vi "___rate scan pruebas.vi"(6 "T Ventana":u32 format="%x", 7 "Espera acceso USB":u32, 8 "error in 2":errorcluster, 9 "Valor buscado scalers (5000)":u16, 10 "Sumador":u8, 11 "ftHandle_in 2":u32) -> (0 "error out 2":errorcluster, 1 "Scaler 3\nTH3,TH4,TH5":u16, 2 "Scaler 2\nTH0,TH1,TH2":u16, 3 "ftHandle_out 2":u32)   [LabVIEW 2009]
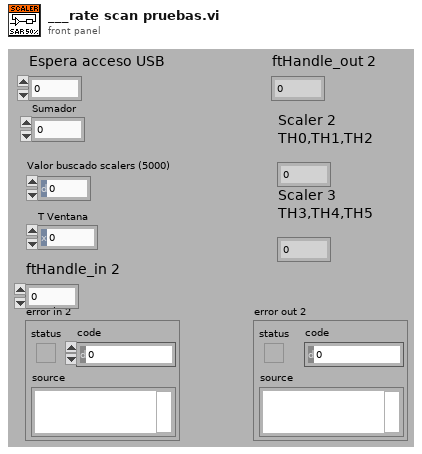
[diagram p1: front panel]
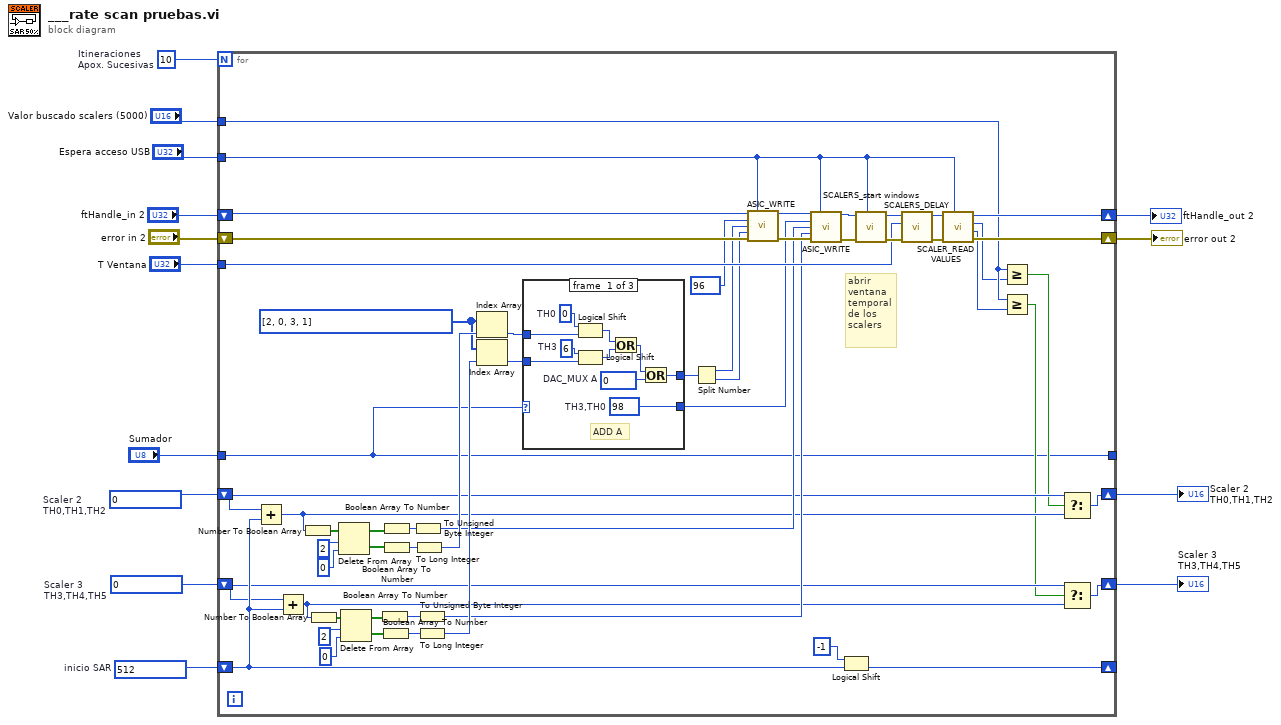
[diagram p0: block diagram]
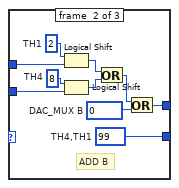
[diagram p2: hidden frame]
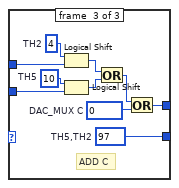
[diagram p3: hidden frame]
diagram:
  w6 = u16 0  # Scaler 3 TH3,TH4,TH5
  w7 = u16 0  # Scaler 2 TH0,TH1,TH2
  w8 = u16 512  # inicio SAR
  w10 = 10  # Itineraciones Apox. Sucesivas
  n1 = for {
    N: w10 -> [_]
    tunnel: "Espera acceso USB" -> [w19]
    tunnel: "T Ventana" -> [w67]
    tunnel: "Valor buscado scalers (5000)" -> [w16]
    shift-right: [w63] -> _
    shift-left: w8 -> [w62]
    shift-right: [w22] -> w4
    shift-left: w7 -> [w29]
    shift-right: [w21] -> w3
    shift-left: w6 -> [w27]
    tunnel: "Sumador" -> [w18]
    shift-right: [w24] -> w2
    shift-left: "ftHandle_in 2" -> [w45]
    shift-right: [w23] -> w1
    shift-left: "error in 2" -> [w44]
    tunnel: [w18] -> _
    w42 = u16[] [2, 0, 3, 1]
    # "abrir ventana temporal de los scalers"
    n2 = Add(x=w29, y=w62) -> (x+y=w28:u16)
    n3 = Add(x=w27, y=w62) -> (x+y=w26:u16)
    n4 = Number To Boolean Array(number=w28) -> (Boolean array=w61:bool[])
    n5 = Number To Boolean Array(number=w26) -> (Boolean array=w60:bool[])
    n6 = Delete From Array(array=w61, length=2, index=0) -> (deleted portion=w54:bool[], array with subset deleted=w59:bool[])
    n7 = Delete From Array(array=w60, length=2, index=0) -> (deleted portion=w52:bool[], array with subset deleted=w53:bool[])
    n8 = Boolean Array To Number(Boolean array=w53) -> (number=w50:u32)
    n9 = Boolean Array To Number(Boolean array=w52) -> (number=w48:u32)
    n10 = Boolean Array To Number(Boolean array=w59) -> (number=w51:u32)
    n11 = Boolean Array To Number(Boolean array=w54) -> (number=w49:u32)
    n12 = To Unsigned Byte Integer(number=w51) -> (unsigned 8bit integer=w33:u8)
    n13 = To Long Integer(number=w49) -> (32bit integer=w47:i32)
    n14 = To Unsigned Byte Integer(number=w50) -> (unsigned 8bit integer=w32:u8)
    n15 = To Long Integer(number=w48) -> (32bit integer=w46:i32)
    n16 = Index Array(array=w42, index=w47) -> (element=w41:u16)
    n17 = Index Array(array=w42, index=w46) -> (element=w40:u16)
    n18 = case shown="0, Default" w18 {
      tunnel: [w79 w89 w99] -> w34
      tunnel: w41 -> [w78 w88 w98]
      tunnel: w40 -> [w77 w87 w97]
      tunnel: [w71 w81 w91] -> w35
      frame #0 {
        w70 = u16 0  # DAC_MUX A
        w75 = i8 6  # TH3
        w76 = i8 0  # TH0
        w79 = u8 98  # TH3,TH0
        # "ADD A"
        n19 = Logical Shift(y=w76, x=w78) -> (x << y=w73:u16)
        n20 = Logical Shift(y=w75, x=w77) -> (x << y=w74:u16)
        n21 = Or(x=w73, y=w74) -> (x .or. y?=w72:u16)
        n22 = Or(x=w72, y=w70) -> (x .or. y?=w71:u16)
      }
      frame #1 {
        w80 = u16 0  # DAC_MUX B
        w85 = i8 8  # TH4
        w86 = i8 2  # TH1
        w89 = u8 99  # TH4,TH1
        # "ADD B"
        n23 = Logical Shift(y=w86, x=w88) -> (x << y=w83:u16)
        n24 = Logical Shift(y=w85, x=w87) -> (x << y=w84:u16)
        n25 = Or(x=w83, y=w84) -> (x .or. y?=w82:u16)
        n26 = Or(x=w82, y=w80) -> (x .or. y?=w81:u16)
      }
      frame #2 {
        w90 = u16 0  # DAC_MUX C
        w95 = i8 10  # TH5
        w96 = i8 4  # TH2
        w99 = u8 97  # TH5,TH2
        # "ADD C"
        n27 = Logical Shift(y=w96, x=w98) -> (x << y=w93:u16)
        n28 = Logical Shift(y=w95, x=w97) -> (x << y=w94:u16)
        n29 = Or(x=w93, y=w94) -> (x .or. y?=w92:u16)
        n30 = Or(x=w92, y=w90) -> (x .or. y?=w91:u16)
      }
    }
    n31 = Split Number(x=w35) -> (hi(x)=w36:u8, lo(x)=w37:u8)
    n32 = call "ASIC_WRITE.vi"("ftHandle_in"=w45, "Espera acceso USB"=w19, "Direccion Registro Asic"=u8 96, "Byte Alto"=w36, "Byte Bajo"=w37, "error in"=w44) -> ("ftHandle_out"=w39:u32, "error out"=w38:errorcluster)  [unwired: 8 in]
    n33 = call "ASIC_WRITE.vi"("ftHandle_in"=w39, "Espera acceso USB"=w19, "Direccion Registro Asic"=w34, "Byte Alto"=w33, "Byte Bajo"=w32, "error in"=w38) -> ("ftHandle_out"=w31:u32, "error out"=w30:errorcluster)  [unwired: 8 in]
    n34 = Logical Shift(y=i8 -1, x=w62) -> (x << y=w63:u16)
    n35 = call "SCALERS_start windows.vi"("Espera acceso USB"=w19, "error in 2"=w30, "ftHandle_in 2"=w31) -> ("error out"=w68:errorcluster, "ftHandle_out"=w69:u32)  [unwired: 7 in]
    n36 = call "SCALERS_DELAY.vi"("error out 2"=w68, "Ventana 2"=w67, "ftHandle_out 2"=w69) -> ("error out"=w65:errorcluster, "ftHandle_out"=w66:u32)  [unwired: 7 in]
    n37 = call "SCALER_READ VALUES.vi"("Espera acceso USB"=w19, "error in"=w65, "ftHandle_in"=w66) -> ("error out"=w23:errorcluster, "Scaler 3"=w17:u16, "Scaler 2"=w15:u16, "ftHandle_out"=w24:u32)  [unwired: 3 in, 2 out]
    n38 = Greater Or Equal?(x=w16, y=w15) -> (x >= y?=w25:bool)
    n39 = Greater Or Equal?(x=w16, y=w17) -> (x >= y?=w20:bool)
    n40 = Select(t=w29, s=w25, f=w28) -> (s? t:f=w22:u16)
    n41 = Select(t=w27, s=w20, f=w26) -> (s? t:f=w21:u16)
  }
  "error out 2" <- w1
  "ftHandle_out 2" <- w2
  "Scaler 2\nTH0,TH1,TH2" <- w4
  "Scaler 3\nTH3,TH4,TH5" <- w3
